vi "Joint_Logic.vi"(0 "Manual_Up":bool, 1 "Manual_Down":bool, 2 "Stow":bool, 3 "Low_Rocket":bool, 4 "Mid_Rocket":bool, 5 "High_Rocket":bool, 6 "Cargo_Ship":bool, 7 "Hatch_Floor":bool, 8 "Depot_Cargo":bool, 9 "Cargo_Floor":bool, 11 "HP_Hatch":bool, 13 "HP_Cargo":bool, 15 "Visited_Disabled":bool) -> (16 "Depot_Cargo_Out":bool, 17 "HP_Cargo_Out":bool, 18 "Manual_Up_Out":bool, 19 "HP_Hatch_Out":bool, 20 "Manual_Down_Out":bool, 21 "Stow_Out":bool, 22 "Low_Rocket_Out":bool, 23 "Mid_Rocket_Out":bool, 24 "High_Rocket_Out":bool, 25 "Cargo_Ship_Out":bool, 26 "Hatch_Floor_Out":bool, 27 "Cargo_Floor_Out":bool)   [LabVIEW 2018]
uses:
  Global_Variables/Elevator_Globals.vi
panel:
  in  "Manual_Up_Scoring":bool
  in  "Manual_Down_Intaking":bool
  in  "Manual_Down_Scoring":bool
  in  "Manual_Up_Intaking":bool
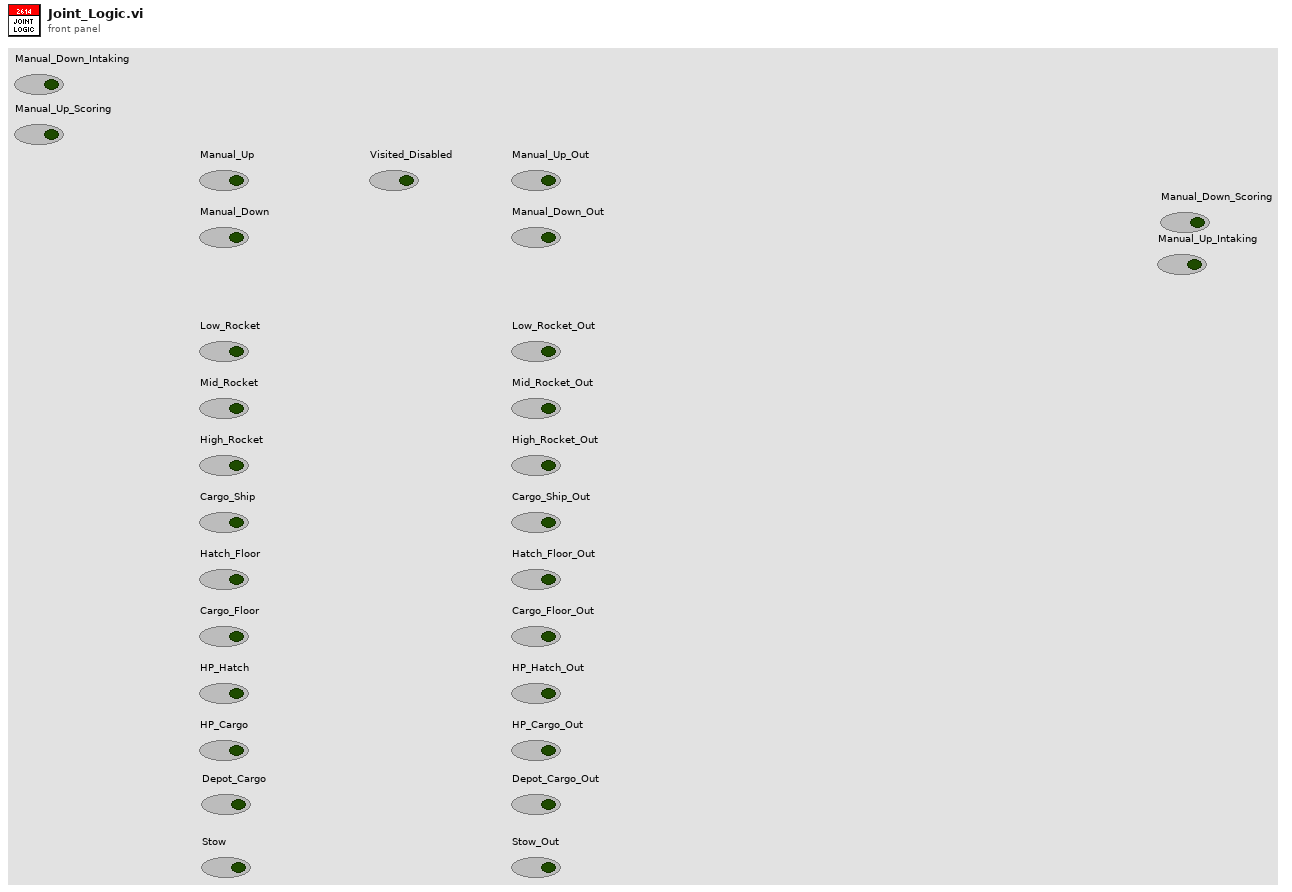
[diagram p1: front panel]
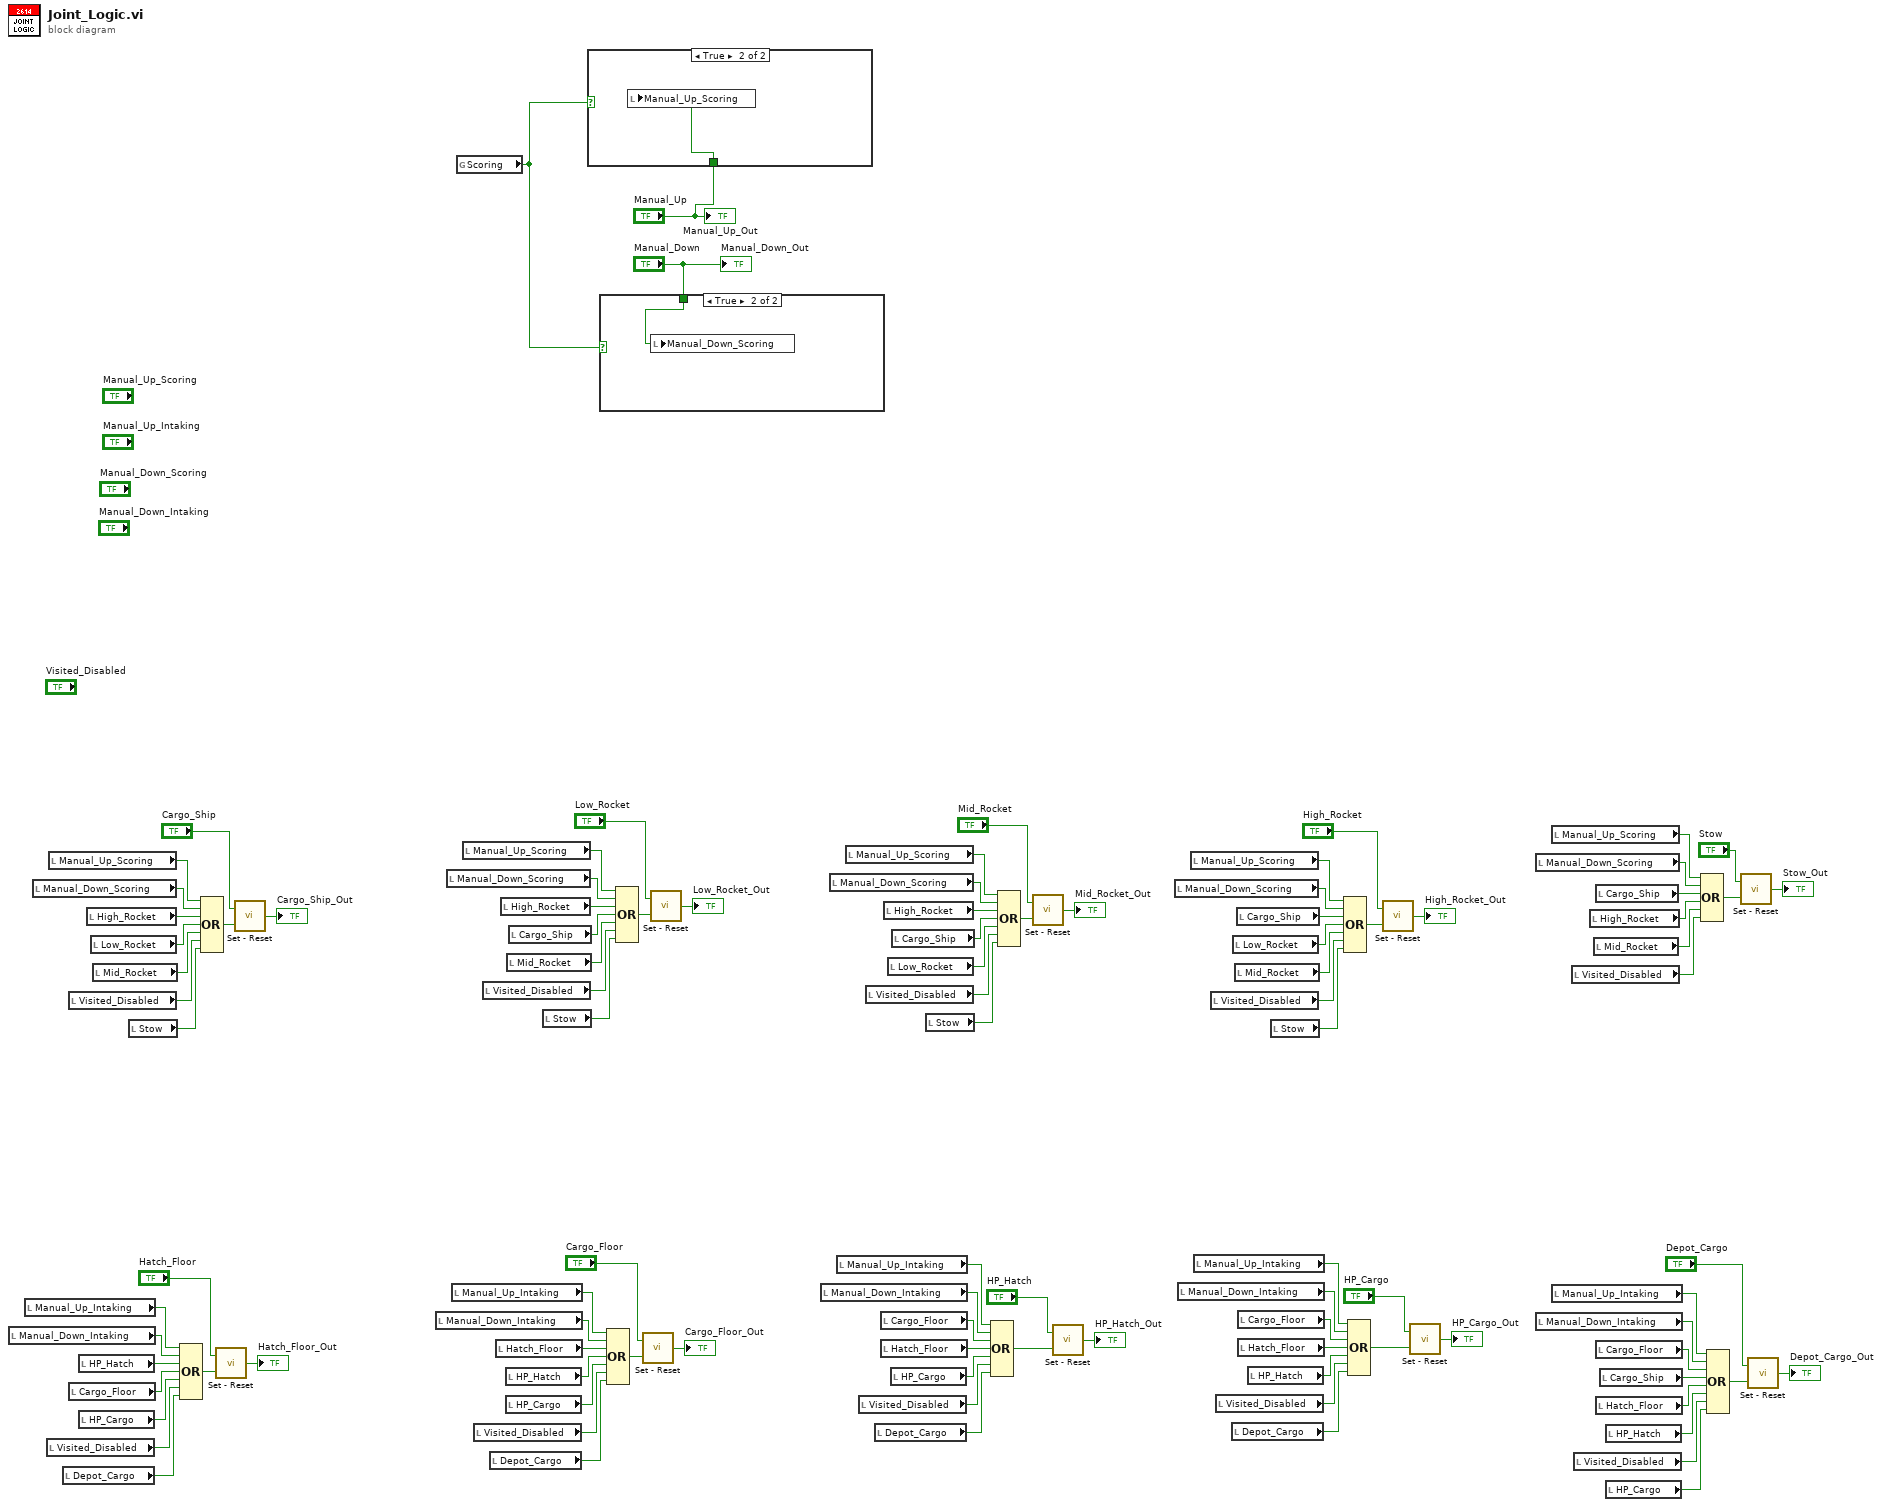
[diagram p0: block diagram]
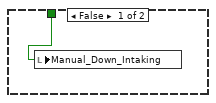
[diagram p2: hidden frame]
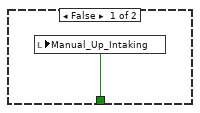
[diagram p3: hidden frame]
diagram:
  n1 = local read "Manual_Down_Intaking"() -> (w75:bool)
  n2 = local read "Manual_Up_Intaking"() -> (w76:bool)
  n3 = local read "Manual_Down_Scoring"() -> (w77:bool)
  n4 = local read "Visited_Disabled"() -> (w81:bool)
  n5 = local read "Manual_Up_Scoring"() -> (w78:bool)
  n6 = local read "Depot_Cargo"() -> (w22:bool)
  n7 = local read "Visited_Disabled"() -> (w79:bool)
  n8 = local read "Cargo_Floor"() -> (w51:bool)
  n9 = local read "HP_Hatch"() -> (w52:bool)
  n10 = local read "HP_Cargo"() -> (w50:bool)
  n11 = local read "High_Rocket"() -> (w59:bool)
  n12 = local read "Low_Rocket"() -> (w58:bool)
  n13 = local read "Mid_Rocket"() -> (w57:bool)
  n14 = local read "Stow"() -> (w4:bool)
  n15 = Compound Arithmetic op=OR(w76, w75, w52, w51, w50, w81, w22) -> (w61:bool)
  n16 = Compound Arithmetic op=OR(w78, w77, w59, w58, w57, w79, w4) -> (w93:bool)
  n17 = call "Set - Reset.vi"("Reset"=w61, "Set"="Hatch_Floor") -> ("Output"=→"Hatch_Floor_Out":bool)
  n18 = call "Set - Reset.vi"("Reset"=w93, "Set"="Cargo_Ship") -> ("Output"=→"Cargo_Ship_Out":bool)
  n19 = local read "Manual_Down_Intaking"() -> (w69:bool)
  n20 = local read "Manual_Down_Scoring"() -> (w73:bool)
  n21 = local read "Manual_Up_Intaking"() -> (w70:bool)
  n22 = global read "Elevator_Globals.vi" "Scoring"() -> (w3:bool)
  n23 = local read "Manual_Up_Scoring"() -> (w74:bool)
  n24 = local read "Visited_Disabled"() -> (w84:bool)
  n25 = local read "Visited_Disabled"() -> (w80:bool)
  n26 = local read "Depot_Cargo"() -> (w23:bool)
  n27 = local read "Hatch_Floor"() -> (w45:bool)
  n28 = local read "High_Rocket"() -> (w56:bool)
  n29 = local read "HP_Hatch"() -> (w44:bool)
  n30 = local read "HP_Cargo"() -> (w43:bool)
  n31 = local read "Mid_Rocket"() -> (w54:bool)
  n32 = local read "Cargo_Ship"() -> (w55:bool)
  n33 = local read "Stow"() -> (w5:bool)
  n34 = case shown="True" w3 {
    tunnel: "Manual_Up" -> [w104 w105]
    frame False {
      n35 = local write "Manual_Up_Intaking"(w104) -> ()
    }
    frame True {
      n36 = local write "Manual_Up_Scoring"(w105) -> ()
    }
  }
  n37 = case shown="True" w3 {
    tunnel: "Manual_Down" -> [w106 w107]
    frame False {
      n38 = local write "Manual_Down_Intaking"(w106) -> ()
    }
    frame True {
      n39 = local write "Manual_Down_Scoring"(w107) -> ()
    }
  }
  n40 = Compound Arithmetic op=OR(w70, w69, w45, w44, w43, w84, w23) -> (w83:bool)
  n41 = Compound Arithmetic op=OR(w74, w73, w56, w55, w54, w80, w5) -> (w62:bool)
  n42 = call "Set - Reset.vi"("Reset"=w83, "Set"="Cargo_Floor") -> ("Output"=→"Cargo_Floor_Out":bool)
  n43 = call "Set - Reset.vi"("Reset"=w62, "Set"="Low_Rocket") -> ("Output"=→"Low_Rocket_Out":bool)
  n44 = local read "Manual_Down_Intaking"() -> (w65:bool)
  n45 = local read "Manual_Down_Scoring"() -> (w71:bool)
  n46 = local read "Manual_Up_Intaking"() -> (w66:bool)
  n47 = local read "Manual_Up_Scoring"() -> (w72:bool)
  n48 = local read "Visited_Disabled"() -> (w88:bool)
  n49 = local read "Visited_Disabled"() -> (w82:bool)
  n50 = local read "Depot_Cargo"() -> (w24:bool)
  n51 = local read "Cargo_Floor"() -> (w39:bool)
  n52 = local read "Hatch_Floor"() -> (w38:bool)
  n53 = local read "High_Rocket"() -> (w49:bool)
  n54 = local read "Low_Rocket"() -> (w47:bool)
  n55 = local read "HP_Cargo"() -> (w37:bool)
  n56 = local read "Cargo_Ship"() -> (w48:bool)
  n57 = local read "Stow"() -> (w6:bool)
  n58 = Compound Arithmetic op=OR(w66, w65, w39, w38, w37, w88, w24) -> (w90:bool)
  n59 = Compound Arithmetic op=OR(w72, w71, w49, w48, w47, w82, w6) -> (w60:bool)
  n60 = call "Set - Reset.vi"("Reset"=w60, "Set"="Mid_Rocket") -> ("Output"=→"Mid_Rocket_Out":bool)
  n61 = call "Set - Reset.vi"("Reset"=w90, "Set"="HP_Hatch") -> ("Output"=→"HP_Hatch_Out":bool)
  n62 = local read "Manual_Down_Scoring"() -> (w67:bool)
  n63 = local read "Manual_Down_Intaking"() -> (w63:bool)
  n64 = local read "Manual_Up_Scoring"() -> (w68:bool)
  n65 = local read "Manual_Up_Intaking"() -> (w64:bool)
  n66 = local read "Visited_Disabled"() -> (w86:bool)
  n67 = local read "Visited_Disabled"() -> (w91:bool)
  n68 = local read "Depot_Cargo"() -> (w25:bool)
  n69 = local read "Low_Rocket"() -> (w41:bool)
  n70 = local read "Mid_Rocket"() -> (w40:bool)
  n71 = local read "Cargo_Ship"() -> (w42:bool)
  n72 = local read "Cargo_Floor"() -> (w34:bool)
  n73 = local read "Hatch_Floor"() -> (w35:bool)
  n74 = local read "HP_Hatch"() -> (w36:bool)
  n75 = local read "Stow"() -> (w7:bool)
  n76 = Compound Arithmetic op=OR(w68, w67, w42, w41, w40, w86, w7) -> (w85:bool)
  n77 = Compound Arithmetic op=OR(w64, w63, w34, w35, w36, w91, w25) -> (w95:bool)
  n78 = call "Set - Reset.vi"("Reset"=w85, "Set"="High_Rocket") -> ("Output"=→"High_Rocket_Out":bool)
  n79 = call "Set - Reset.vi"("Reset"=w95, "Set"="HP_Cargo") -> ("Output"=→"HP_Cargo_Out":bool)
  n80 = local read "Manual_Down_Scoring"() -> (w14:bool)
  n81 = local read "Manual_Down_Intaking"() -> (w29:bool)
  n82 = local read "Manual_Up_Scoring"() -> (w15:bool)
  n83 = local read "Manual_Up_Intaking"() -> (w28:bool)
  n84 = local read "Visited_Disabled"() -> (w16:bool)
  n85 = local read "Visited_Disabled"() -> (w27:bool)
  n86 = local read "High_Rocket"() -> (w12:bool)
  n87 = local read "Mid_Rocket"() -> (w13:bool)
  n88 = local read "Cargo_Ship"() -> (w11:bool)
  n89 = local read "Cargo_Floor"() -> (w33:bool)
  n90 = local read "Hatch_Floor"() -> (w31:bool)
  n91 = local read "Cargo_Ship"() -> (w32:bool)
  n92 = local read "HP_Hatch"() -> (w30:bool)
  n93 = local read "HP_Cargo"() -> (w21:bool)
  n94 = Compound Arithmetic op=OR(w15, w14, w11, w12, w13, w16) -> (w9:bool)
  n95 = Compound Arithmetic op=OR(w28, w29, w33, w32, w31, w30, w27, w21) -> (w26:bool)
  n96 = call "Set - Reset.vi"("Reset"=w9, "Set"="Stow") -> ("Output"=→"Stow_Out":bool)
  n97 = call "Set - Reset.vi"("Reset"=w26, "Set"="Depot_Cargo") -> ("Output"=→"Depot_Cargo_Out":bool)
  "Manual_Up_Out" <- "Manual_Up"
  "Manual_Down_Out" <- "Manual_Down"
